vi "Prickle a structure towards its boundary.vi"(10 "Prickle Distance (Cartesian)":dbl(slide) scale=0.0..0.5, 11 "Input Structure":T1={"Structure Name"="Gamma8_64atom", "Lattice vector a"=[13.21796569573, 0.0, 0.0], "Lattice vector b"=[0.0, 13.21796569573, 0.0], "Lattice vector c"=[0.0, 0.0, 13.21796569573], "Atoms Array"=[{"Atom Name"="Cd", "Positions (Direct)"=[[0.0, 0.0, 0.0], [0.0, 0.0, 0.5], [0.0, 0.5, 0.0], [0.0, 0.5, 0.5], [0.5, 0.0, 0.0], [0.5, 0.0, 0.5], [0.5, 0.5, 0.0], [0.5, 0.5, 0.5], [0.0, 0.25, 0.25], [0.0, 0.25, 0.75], [0.0, 0.75, 0.25], [0.0, 0.75, 0.75], [0.5, 0.25, 0.25], [0.5, 0.25, 0.75], [0.5, 0.75, 0.25], [0.5, 0.75, 0.75], [0.25, 0.0, 0.25], [0.25, 0.0, 0.75], [0.25, 0.5, 0.25], [0.25, 0.5, 0.75], [0.75, 0.0, 0.25], [0.75, 0.0, 0.75], [0.75, 0.5, 0.25], [0.75, 0.5, 0.75], [0.25, 0.25, 0.0], [0.25, 0.25, 0.5], [0.25, 0.75, 0.0], [0.25, 0.75, 0.5], [0.75, 0.25, 0.0], [0.75, 0.25, 0.5], [0.75, 0.75, 0.0], [0.75, 0.75, 0.5]], "Positions (Cartesian)"=[[0.0, 0.0, 0.0], [0.0, 0.0, 6.608982847865], [0.0, 6.608982847865, 0.0], [0.0, 6.608982847865, 6.608982847865], [6.608982847865, 0.0, 0.0], [6.608982847865, 0.0, 6.608982847865], [6.608982847865, 6.608982847865, 0.0], [6.608982847865, 6.608982847865, 6.608982847865], [0.0, 3.3044914239325, 3.3044914239325], [0.0, 3.3044914239325, 9.913474271797499], [0.0, 9.913474271797499, 3.3044914239325], [0.0, 9.913474271797499, 9.913474271797499], [6.608982847865, 3.3044914239325, 3.3044914239325], [6.608982847865, 3.3044914239325, 9.913474271797499], [6.608982847865, 9.913474271797499, 3.3044914239325], [6.608982847865, 9.913474271797499, 9.913474271797499], [3.3044914239325, 0.0, 3.3044914239325], [3.3044914239325, 0.0, 9.913474271797499], [3.3044914239325, 6.608982847865, 3.3044914239325], [3.3044914239325, 6.608982847865, 9.913474271797499], [9.913474271797499, 0.0, 3.3044914239325], [9.913474271797499, 0.0, 9.913474271797499], [9.913474271797499, 6.608982847865, 3.3044914239325], [9.913474271797499, 6.608982847865, 9.913474271797499], [3.3044914239325, 3.3044914239325, 0.0], [3.3044914239325, 3.3044914239325, 6.608982847865], [3.3044914239325, 9.913474271797499, 0.0], [3.3044914239325, 9.913474271797499, 6.608982847865], [9.913474271797499, 3.3044914239325, 0.0], [9.913474271797499, 3.3044914239325, 6.608982847865], [9.913474271797499, 9.913474271797499, 0.0], [9.913474271797499, 9.913474271797499, 6.608982847865]]}, {"Atom Name"="Te", "Positions (Direct)"=[[0.125, 0.125, 0.125], [0.125, 0.125, 0.625], [0.125, 0.625, 0.125], [0.125, 0.625, 0.625], [0.625, 0.125, 0.125], [0.625, 0.125, 0.625], [0.625, 0.625, 0.125], [0.625, 0.625, 0.625], [0.375, 0.375, 0.125], [0.375, 0.375, 0.625], [0.375, 0.875, 0.125], [0.375, 0.875, 0.625], [0.875, 0.375, 0.125], [0.875, 0.375, 0.625], [0.875, 0.875, 0.125], [0.875, 0.875, 0.625], [0.375, 0.125, 0.375], [0.375, 0.125, 0.875], [0.375, 0.625, 0.375], [0.375, 0.625, 0.875], [0.875, 0.125, 0.375], [0.875, 0.125, 0.875], [0.875, 0.625, 0.375], [0.875, 0.625, 0.875], [0.125, 0.375, 0.375], [0.125, 0.375, 0.875], [0.125, 0.875, 0.375], [0.125, 0.875, 0.875], [0.625, 0.375, 0.375], [0.625, 0.375, 0.875], [0.625, 0.875, 0.375], [0.625, 0.875, 0.875]], "Positions (Cartesian)"=[[1.65224571196625, 1.65224571196625, 1.65224571196625], [1.65224571196625, 1.65224571196625, 8.261228559831249], [1.65224571196625, 8.261228559831249, 1.65224571196625], [1.65224571196625, 8.261228559831249, 8.261228559831249], [8.261228559831249, 1.65224571196625, 1.65224571196625], [8.261228559831249, 1.65224571196625, 8.261228559831249], [8.261228559831249, 8.261228559831249, 1.65224571196625], [8.261228559831249, 8.261228559831249, 8.261228559831249], [4.9567371358987495, 4.9567371358987495, 1.65224571196625], [4.9567371358987495, 4.9567371358987495, 8.261228559831249], [4.9567371358987495, 11.56571998376375, 1.65224571196625], [4.9567371358987495, 11.56571998376375, 8.261228559831249], [11.56571998376375, 4.9567371358987495, 1.65224571196625], [11.56571998376375, 4.9567371358987495, 8.261228559831249], [11.56571998376375, 11.56571998376375, 1.65224571196625], [11.56571998376375, 11.56571998376375, 8.261228559831249], [4.9567371358987495, 1.65224571196625, 4.9567371358987495], [4.9567371358987495, 1.65224571196625, 11.56571998376375], [4.9567371358987495, 8.261228559831249, 4.9567371358987495], [4.9567371358987495, 8.261228559831249, 11.56571998376375], [11.56571998376375, 1.65224571196625, 4.9567371358987495], [11.56571998376375, 1.65224571196625, 11.56571998376375], [11.56571998376375, 8.261228559831249, 4.9567371358987495], [11.56571998376375, 8.261228559831249, 11.56571998376375], [1.65224571196625, 4.9567371358987495, 4.9567371358987495], [1.65224571196625, 4.9567371358987495, 11.56571998376375], [1.65224571196625, 11.56571998376375, 4.9567371358987495], [1.65224571196625, 11.56571998376375, 11.56571998376375], [8.261228559831249, 4.9567371358987495, 4.9567371358987495], [8.261228559831249, 4.9567371358987495, 11.56571998376375], [8.261228559831249, 11.56571998376375, 4.9567371358987495], [8.261228559831249, 11.56571998376375, 11.56571998376375]]}], "# of atoms"=64}) -> (3 "Prickled Structure":T1={"Structure Name"="Gamma8_64atom", "Lattice vector a"=[13.21796569573, 0.0, 0.0], "Lattice vector b"=[0.0, 13.21796569573, 0.0], "Lattice vector c"=[0.0, 0.0, 13.21796569573], "Atoms Array"=[{"Atom Name"="Cd", "Positions (Direct)"=[[0.0, 0.0, 0.0], [0.0, 0.0, 0.5], [0.0, 0.5, 0.0], [0.0, 0.5, 0.5], [0.5, 0.0, 0.0], [0.5, 0.0, 0.5], [0.5, 0.5, 0.0], [0.5, 0.5, 0.5], [0.0, 0.25, 0.25], [0.0, 0.25, 0.75], [0.0, 0.75, 0.25], [0.0, 0.75, 0.75], [0.5, 0.25, 0.25], [0.5, 0.25, 0.75], [0.5, 0.75, 0.25], [0.5, 0.75, 0.75], [0.25, 0.0, 0.25], [0.25, 0.0, 0.75], [0.25, 0.5, 0.25], [0.25, 0.5, 0.75], [0.75, 0.0, 0.25], [0.75, 0.0, 0.75], [0.75, 0.5, 0.25], [0.75, 0.5, 0.75], [0.25, 0.25, 0.0], [0.25, 0.25, 0.5], [0.25, 0.75, 0.0], [0.25, 0.75, 0.5], [0.75, 0.25, 0.0], [0.75, 0.25, 0.5], [0.75, 0.75, 0.0], [0.75, 0.75, 0.5]], "Positions (Cartesian)"=[[0.0, 0.0, 0.0], [0.0, 0.0, 6.608982847865], [0.0, 6.608982847865, 0.0], [0.0, 6.608982847865, 6.608982847865], [6.608982847865, 0.0, 0.0], [6.608982847865, 0.0, 6.608982847865], [6.608982847865, 6.608982847865, 0.0], [6.608982847865, 6.608982847865, 6.608982847865], [0.0, 3.3044914239325, 3.3044914239325], [0.0, 3.3044914239325, 9.913474271797499], [0.0, 9.913474271797499, 3.3044914239325], [0.0, 9.913474271797499, 9.913474271797499], [6.608982847865, 3.3044914239325, 3.3044914239325], [6.608982847865, 3.3044914239325, 9.913474271797499], [6.608982847865, 9.913474271797499, 3.3044914239325], [6.608982847865, 9.913474271797499, 9.913474271797499], [3.3044914239325, 0.0, 3.3044914239325], [3.3044914239325, 0.0, 9.913474271797499], [3.3044914239325, 6.608982847865, 3.3044914239325], [3.3044914239325, 6.608982847865, 9.913474271797499], [9.913474271797499, 0.0, 3.3044914239325], [9.913474271797499, 0.0, 9.913474271797499], [9.913474271797499, 6.608982847865, 3.3044914239325], [9.913474271797499, 6.608982847865, 9.913474271797499], [3.3044914239325, 3.3044914239325, 0.0], [3.3044914239325, 3.3044914239325, 6.608982847865], [3.3044914239325, 9.913474271797499, 0.0], [3.3044914239325, 9.913474271797499, 6.608982847865], [9.913474271797499, 3.3044914239325, 0.0], [9.913474271797499, 3.3044914239325, 6.608982847865], [9.913474271797499, 9.913474271797499, 0.0], [9.913474271797499, 9.913474271797499, 6.608982847865]]}, {"Atom Name"="Te", "Positions (Direct)"=[[0.125, 0.125, 0.125], [0.125, 0.125, 0.625], [0.125, 0.625, 0.125], [0.125, 0.625, 0.625], [0.625, 0.125, 0.125], [0.625, 0.125, 0.625], [0.625, 0.625, 0.125], [0.625, 0.625, 0.625], [0.375, 0.375, 0.125], [0.375, 0.375, 0.625], [0.375, 0.875, 0.125], [0.375, 0.875, 0.625], [0.875, 0.375, 0.125], [0.875, 0.375, 0.625], [0.875, 0.875, 0.125], [0.875, 0.875, 0.625], [0.375, 0.125, 0.375], [0.375, 0.125, 0.875], [0.375, 0.625, 0.375], [0.375, 0.625, 0.875], [0.875, 0.125, 0.375], [0.875, 0.125, 0.875], [0.875, 0.625, 0.375], [0.875, 0.625, 0.875], [0.125, 0.375, 0.375], [0.125, 0.375, 0.875], [0.125, 0.875, 0.375], [0.125, 0.875, 0.875], [0.625, 0.375, 0.375], [0.625, 0.375, 0.875], [0.625, 0.875, 0.375], [0.625, 0.875, 0.875]], "Positions (Cartesian)"=[[1.65224571196625, 1.65224571196625, 1.65224571196625], [1.65224571196625, 1.65224571196625, 8.261228559831249], [1.65224571196625, 8.261228559831249, 1.65224571196625], [1.65224571196625, 8.261228559831249, 8.261228559831249], [8.261228559831249, 1.65224571196625, 1.65224571196625], [8.261228559831249, 1.65224571196625, 8.261228559831249], [8.261228559831249, 8.261228559831249, 1.65224571196625], [8.261228559831249, 8.261228559831249, 8.261228559831249], [4.9567371358987495, 4.9567371358987495, 1.65224571196625], [4.9567371358987495, 4.9567371358987495, 8.261228559831249], [4.9567371358987495, 11.56571998376375, 1.65224571196625], [4.9567371358987495, 11.56571998376375, 8.261228559831249], [11.56571998376375, 4.9567371358987495, 1.65224571196625], [11.56571998376375, 4.9567371358987495, 8.261228559831249], [11.56571998376375, 11.56571998376375, 1.65224571196625], [11.56571998376375, 11.56571998376375, 8.261228559831249], [4.9567371358987495, 1.65224571196625, 4.9567371358987495], [4.9567371358987495, 1.65224571196625, 11.56571998376375], [4.9567371358987495, 8.261228559831249, 4.9567371358987495], [4.9567371358987495, 8.261228559831249, 11.56571998376375], [11.56571998376375, 1.65224571196625, 4.9567371358987495], [11.56571998376375, 1.65224571196625, 11.56571998376375], [11.56571998376375, 8.261228559831249, 4.9567371358987495], [11.56571998376375, 8.261228559831249, 11.56571998376375], [1.65224571196625, 4.9567371358987495, 4.9567371358987495], [1.65224571196625, 4.9567371358987495, 11.56571998376375], [1.65224571196625, 11.56571998376375, 4.9567371358987495], [1.65224571196625, 11.56571998376375, 11.56571998376375], [8.261228559831249, 4.9567371358987495, 4.9567371358987495], [8.261228559831249, 4.9567371358987495, 11.56571998376375], [8.261228559831249, 11.56571998376375, 4.9567371358987495], [8.261228559831249, 11.56571998376375, 11.56571998376375]]}], "# of atoms"=64})   [LabVIEW 2010]
uses:
  <vilib>/Analysis/baseanly.llb/Real Dot Product.vi
  <vilib>/Analysis/_algsub.llb/Real Vector Norm.vi
  <vilib>/Analysis/NI_AALBase.lvlib
  <vilib>/Analysis/NI_AALPro.lvlib
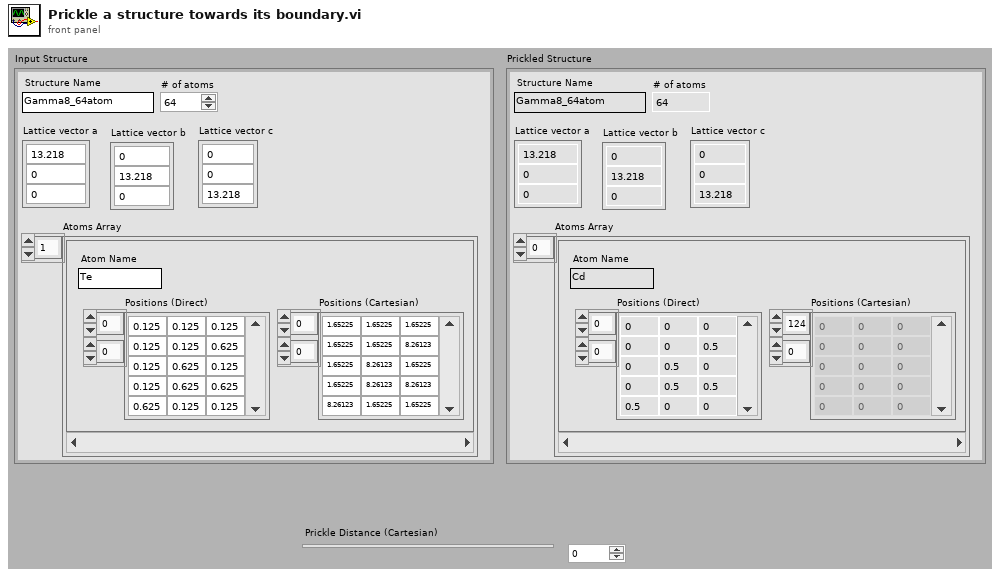
[diagram p1: front panel]
types:
  T1 = cluster{"Structure Name":string, "Lattice vector a":dbl[], "Lattice vector b":dbl[], "Lattice vector c":dbl[], "Atoms Array":cluster{"Atom Name":string, "Positions (Direct)":dbl[][], "Positions (Cartesian)":dbl[][]}[], "# of atoms":i32}
  T2 = cluster{"Atom Name":string, "Positions (Direct)":dbl[][], "Positions (Cartesian)":dbl[][]}[]
  T3 = cluster{"Atom Name":string, "Positions (Direct)":dbl[][], "Positions (Cartesian)":dbl[][]}
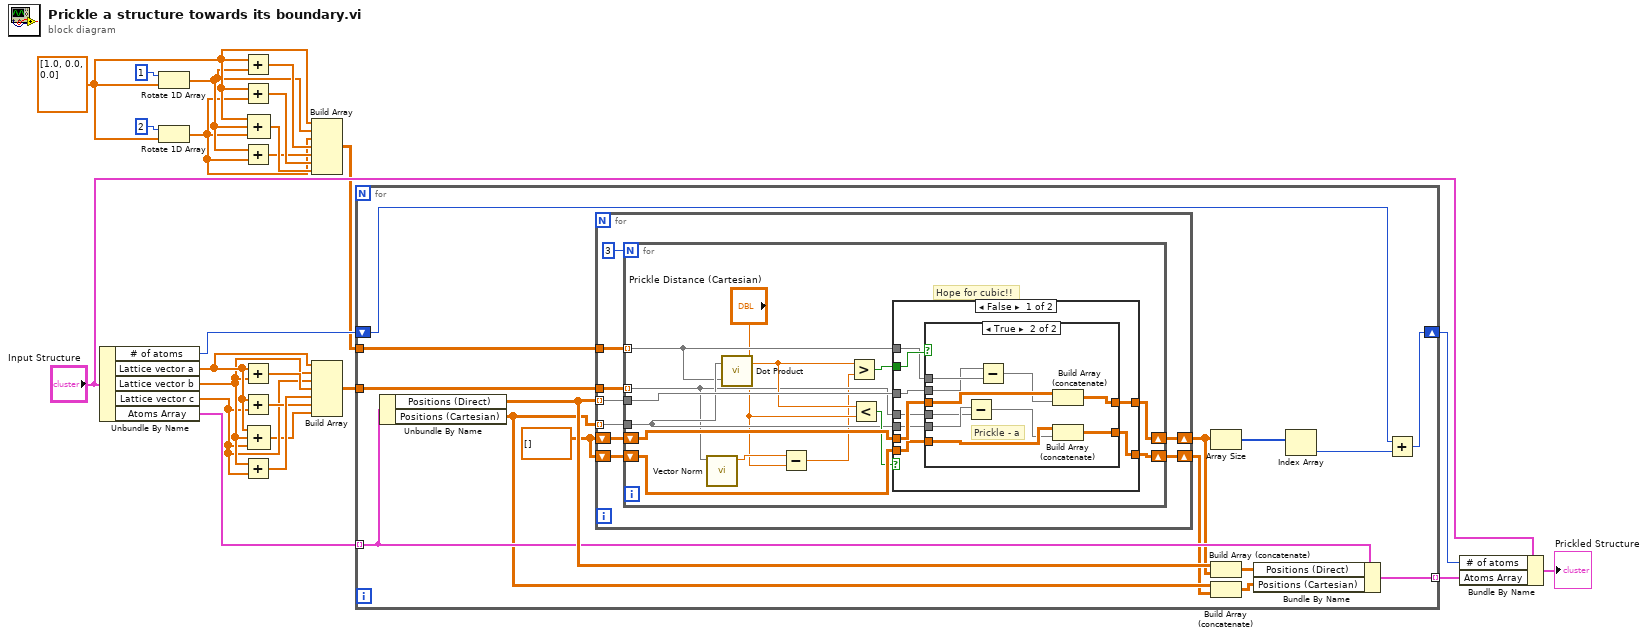
[diagram p0: block diagram]
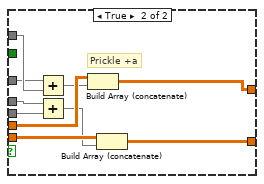
[diagram p3: hidden frame]
diagram:
  w6 = dbl[] [1.0, 0.0, 0.0]
  n1 = Unbundle By Name("Input Structure") -> ("# of atoms"=w19:i32, "Lattice vector a"=w14:dbl[], "Lattice vector b"=w13:dbl[], "Lattice vector c"=w12:dbl[], "Atoms Array"=w24:T2)
  n2 = Rotate 1D Array(1:w6, 2:1 ("n")) -> (0:w5:dbl[])
  n3 = Rotate 1D Array(1:w6, 2:2 ("n")) -> (0:w4:dbl[])
  n4 = Add(x=w6, y=w5) -> (x+y=w7:dbl[])
  n5 = Add(x=w6, y=w4) -> (x+y=w9:dbl[])
  n6 = Add(x=w5, y=w4) -> (x+y=w8:dbl[])
  n7 = Add(x=w14, y=w13) -> (x+y=w17:dbl[])
  n8 = Add(x=w14, y=w12) -> (x+y=w15:dbl[])
  n9 = Add(x=w13, y=w12) -> (x+y=w16:dbl[])
  n10 = Compound Arithmetic op=unknown(w6, w5, w4) -> (w10:dbl[])
  n11 = Compound Arithmetic op=ADD(w14, w13, w12) -> (w11:dbl[])
  n12 = Build Array(w6, w5, w4, w7, w8, w9, w10) -> (w1:dbl[][])
  n13 = Build Array(w14, w13, w12, w17, w16, w15, w11) -> (w23:dbl[][])
  n14 = for {
    tunnel: w24 -> [w37] mode=indexing
    tunnel: w23 -> [w39]
    tunnel: [w35] -> w20 mode=indexing
    shift-right: [w29] -> w18
    shift-left: w19 -> [w33]
    tunnel: w1 -> [w25]
    w34 = dbl[][] []
    n15 = Unbundle By Name(w37) -> ("Positions (Direct)"=w38:dbl[][], "Positions (Cartesian)"=w28:dbl[][])
    n16 = for {
      tunnel: w38 -> [w47] mode=indexing
      tunnel: w39 -> [w48]
      shift-right: [w46] -> w32
      shift-left: w34 -> [w45]
      shift-right: [w42] -> w27
      shift-left: w34 -> [w44]
      tunnel: w28 -> [w43] mode=indexing
      tunnel: w25 -> [w41]
      n17 = for {
        N: 3 -> [_]
        tunnel: w48 -> [w52] mode=indexing
        tunnel: w47 -> [w62]
        shift-right: [w61] -> w46
        shift-left: w45 -> [w60]
        shift-right: [w58] -> w42
        shift-left: w44 -> [w59]
        tunnel: w43 -> [w55]
        tunnel: w41 -> [w54] mode=indexing
        # "Hope for cubic!!"
        n18 = call-poly <vilib>:"Vector Norm.vi"("Input Vector"=w52) -> ("norm"=w51:dbl)  [unwired: 9 in, 1 out]
        n19 = call-poly <vilib>:"Dot Product.vi"("Y Vector"=w54, "X Vector"=w55) -> ("X * Y"=w53:dbl)  [unwired: 1 out]
        n20 = Subtract(x=w51, y="Prickle Distance (Cartesian)") -> (x-y=w49:dbl)
        n21 = Greater?(x=w53, y=w49) -> (0:w57:bool)
        n22 = Less?(x=w53, y="Prickle Distance (Cartesian)") -> (x < y?=w56:bool)
        n23 = case shown="False" w56 {
          tunnel: w57 -> [w71 _]
          tunnel: w62 -> [w69 w85]
          tunnel: [w68 w93] -> w61
          tunnel: w60 -> [w70 w92]
          tunnel: w59 -> [w67 w90]
          tunnel: [w66 w91] -> w58
          tunnel: w52 -> [w64 w89]
          tunnel: w55 -> [w65 w88]
          tunnel: w54 -> [w63 w86]
          frame False {
            n24 = case shown="True" w71 {
              tunnel: w70 -> [w73 w83]
              tunnel: w69 -> [_ w75]
              tunnel: [w73 w82] -> w68
              tunnel: w67 -> [w72 w81]
              tunnel: [w72 w80] -> w66
              tunnel: w65 -> [_ w79]
              tunnel: w64 -> [_ w78]
              tunnel: w63 -> [_ w76]
              frame False {
                # "No prickle"
              }
              frame True {
                # "Prickle - a"
                n25 = Subtract(x=w79, y=w78) -> (x-y=w77:dbl[])
                n26 = Subtract(x=w75, y=w76) -> (x-y=w74:dbl[])
                n27 = Build Array (concatenate)(w83, w74) -> (w82:dbl[][])
                n28 = Build Array (concatenate)(w81, w77) -> (w80:dbl[][])
              }
            }
          }
          frame True {
            # "Prickle +a"
            n29 = Add(x=w85, y=w86) -> (x+y=w84:dbl[])
            n30 = Add(x=w89, y=w88) -> (x+y=w87:dbl[])
            n31 = Build Array (concatenate)(w92, w84) -> (w93:dbl[][])
            n32 = Build Array (concatenate)(w90, w87) -> (w91:dbl[][])
          }
        }
      }
    }
    n33 = Array Size(array=w32) -> (size(s)=w31:i32[])
    n34 = Build Array (concatenate)(w38, w32) -> (w36:dbl[][])
    n35 = Build Array (concatenate)(w28, w27) -> (w26:dbl[][])
    n36 = Bundle By Name(cluster=w37, "Positions (Direct)"=w36, "Positions (Cartesian)"=w26) -> (w35:T3)
    n37 = Index Array(array=w31) -> (element=w30:i32)  [unwired: 1 in]
    n38 = Add(x=w33, y=w30) -> (x+y=w29:i32)
  }
  n39 = Bundle By Name(cluster="Input Structure", "# of atoms"=w18, "Atoms Array"=w20) -> (→"Prickled Structure":T1)
